vi "Protocol.Command.Main.vi"(8 "Error":errorcluster, 11 "J1939 Main Configuration":T1) -> (0 "error out":errorcluster)   [LabVIEW 2015, in "J1939 Addon Engine.lvlib"]
uses:
  J1939 Addon Engine.lvlib
  Types/Protocol.Configuration.ctl
  <vilib>/NI/NIVS Addon Network Comm/Engine/VeriStand Comm.lvclass
  <vilib>/NI/NIVS Inline Async API/_VS Inline Async API/Process/Process.lvclass
  Types/Protocol.Refs.ctl
  Shared/J1939 Utilities/Types/CAN Outgoing Message Cluster.ctl
  Types/Protocol.RQST Lookup Table Reference.ctl
  Types/Protocol.Address Table Reference.ctl
  Types/Protocol.XNET Settings.ctl
  <vilib>/NI/NIVS Inline Async API/_Data Access Engine/Data Access Engine/Types/Read.DVR.ctl
  <vilib>/NI/NIVS Inline Async API/_Data Access Engine/Access Type Classes/Read/Read.lvclass
  <vilib>/NI/NIVS Inline Async API/_Data Access Engine/Data Access Engine/Types/Write.DVR.ctl
  <vilib>/NI/NIVS Inline Async API/_Data Access Engine/Access Type Classes/Write/Write.lvclass
  Types/Protocol.Command.Commands.ctl
  Types/Protocol.Command.Responses.ctl
  <vilib>/NI/NIVS Inline Async API/_Data Access Engine/Access Type Classes/Read/Read.lvclass/Read.ctl
  <vilib>/NI/NIVS Inline Async API/_Data Access Engine/Access Type Classes/Write/Write.lvclass/Write.ctl
  APIs/Host Automation API/Types/DTC_Action.ctl
  <vilib>/NI/NIVS Inline Async API/_VS Inline Async API/Process/Process.lvclass/Process.ctl
  <vilib>/NI/NIVS Inline Async API/_Data Access Engine/Data Access Engine/Methods/Write.Data.vi
  <vilib>/NI/NIVS Inline Async API/_Data Access Engine/Data Access Engine/Methods/Read.Data.vi
  <vilib>/NI/NIVS Inline Async API/_Data Access Engine/Access Type Classes/Write/Write.ProcessData.vi
  <vilib>/NI/NIVS Inline Async API/_VS Inline Async API/Error Handling Process/SubVIs/Error.ConvertArray.vi
  <vilib>/NI/NIVS Inline Async API/_Data Access Engine/Access Type Classes/Read/Read.ProcessData.vi
  APIs/Host Automation API/J1939 Host Automation API.lvlib
  Shared/J1939 Addon Shared.lvlib
  <vilib>/NI VeriStand/Custom Device Tools/Custom Device Utility Library/Custom Device Utility Library.lvlib
  <vilib>/NI/NIVS Inline Async API/_Data Access Engine/Data Access Engine/Data Access Engine.lvclass
  Shared/J1939 Utilities/J1939 Utilities.lvlib
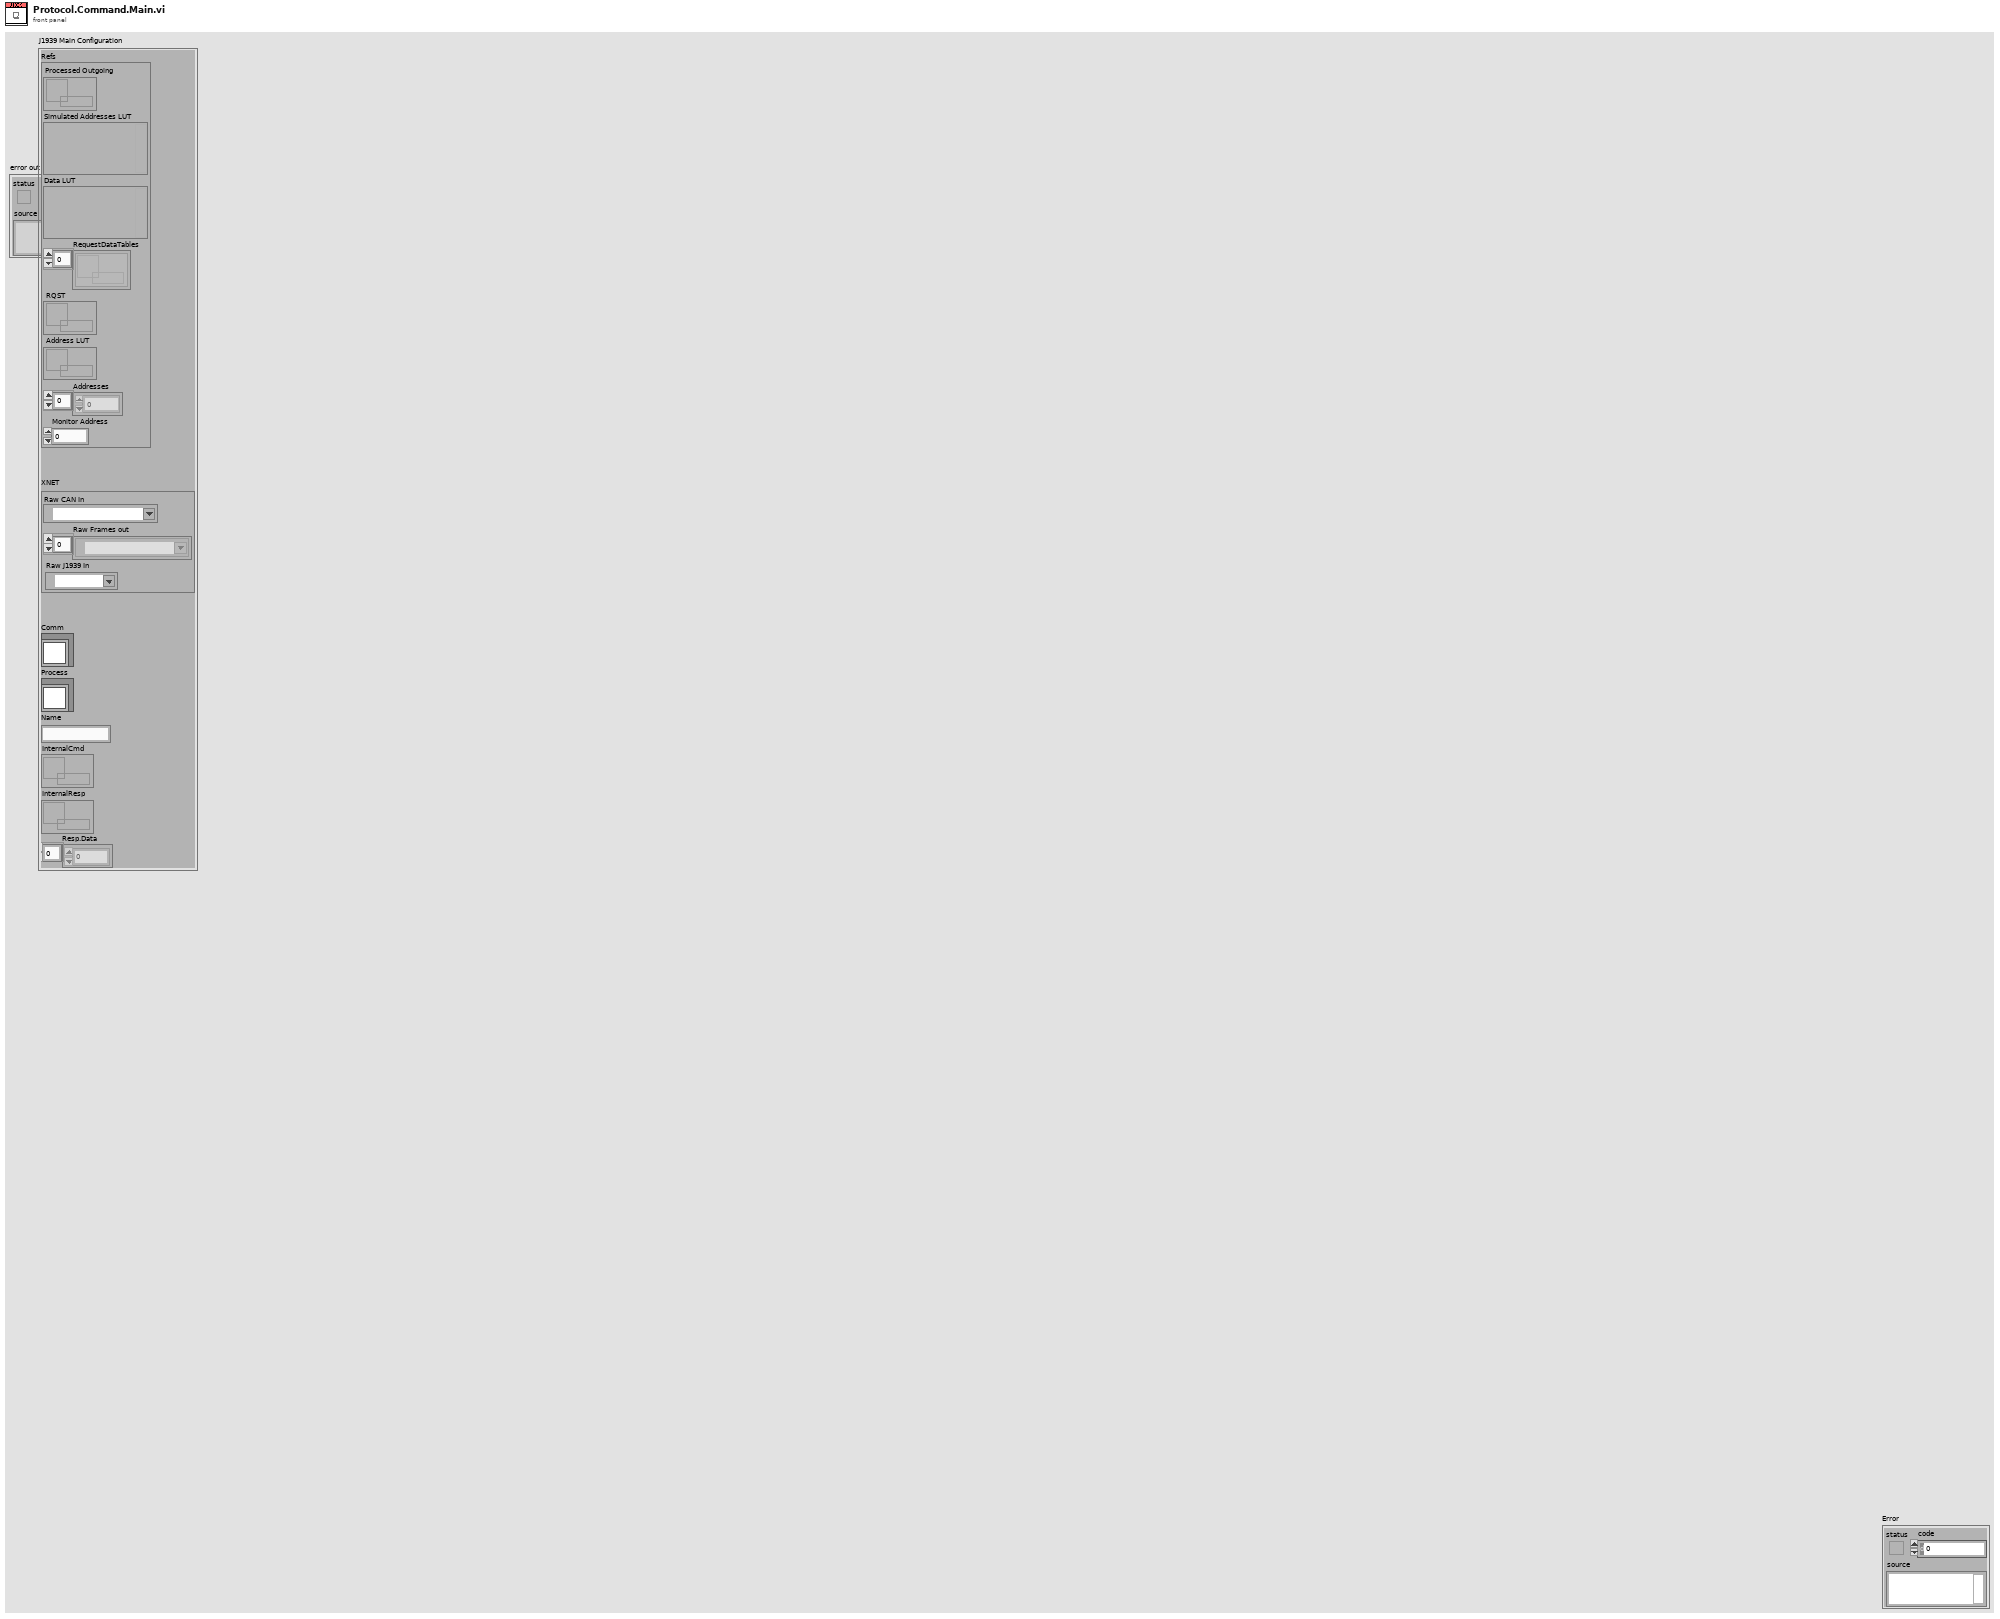
[diagram p1: front panel]
types:
  T1 = typedef "J1939 Addon Engine.lvlib/Protocol.Configuration.ctl" = cluster{"Refs":T2, "XNET":T5, "Comm":refnum<class "VeriStand Comm.lvclass">, "Process":refnum<class "Process.lvclass">, "Name":string, "InternalCmd":T6, "InternalResp":T7, "Resp.Data":dbl[]}
  T2 = typedef "J1939 Addon Engine.lvlib/Protocol.Refs.ctl" = cluster{"Processed Outgoing":refnum<queue>, "Simulated Addresses LUT":variant, "Data LUT":variant, "RequestDataTables":refnum<k33>[], "RQST":T3, "Address LUT":T4, "Addresses":u8[], "Monitor Address":u8}
  T3 = typedef "J1939 Addon Engine.lvlib/Protocol.RQST Lookup Table Reference.ctl" = refnum<data-value>
  T4 = typedef "J1939 Addon Engine.lvlib/Protocol.Address Table Reference.ctl" = refnum<data-value>
  T5 = typedef "J1939 Addon Engine.lvlib/Protocol.XNET Settings.ctl" = cluster{"Raw CAN In":refnum<k21>, "Raw Frames out":refnum<k21>[], "Raw J1939 In":refnum<k21>}
  T6 = typedef "Data Access Engine.lvlib/Data Access Engine.lvclass/Read.DVR.ctl" = refnum<data-value>
  T7 = typedef "Data Access Engine.lvlib/Data Access Engine.lvclass/Write.DVR.ctl" = refnum<data-value>
  T8 = typedef "NI STM.lvlib/TCP Connection Info.ctl" = cluster{"connection ID":refnum<k5>, "meta data":T9[]}
  T9 = typedef "NI STM.lvlib/MetaDataElement.ctl" = string
  T10 = typedef "J1939 Addon Engine.lvlib/Protocol.Command.Responses.ctl" = enum16{"Diagnostic Error Code", "Diagnostic Command Success", "# of DTCs Found", "Request DTC Status"}
  T11 = typedef "J1939 Addon Engine.lvlib/Protocol.Command.Commands.ctl" = enum16{"Diagnostic Command", "Expected DTC", "Address to Query", "DTC Clear Type"}
  T12 = typedef "J1939 Host Automation API.lvlib/DTC_Action.ctl" = enum16{"ALL", "ACTIVE", "INACTIVE"}
  T13 = typedef "J1939 Addon Engine.lvlib/Protocol.Command.States.ctl" = enum8{"Idle", "Refresh Address", "Verify DTCs", "Clear DTCs", "Clear Status Bit", "Clear Error Bit"}
  T14 = typedef "J1939 Host Automation API.lvlib/Verify DTC_Status.ctl" = enum16{"NOT_PRESENT", "ACTIVE", "INACTIVE"}
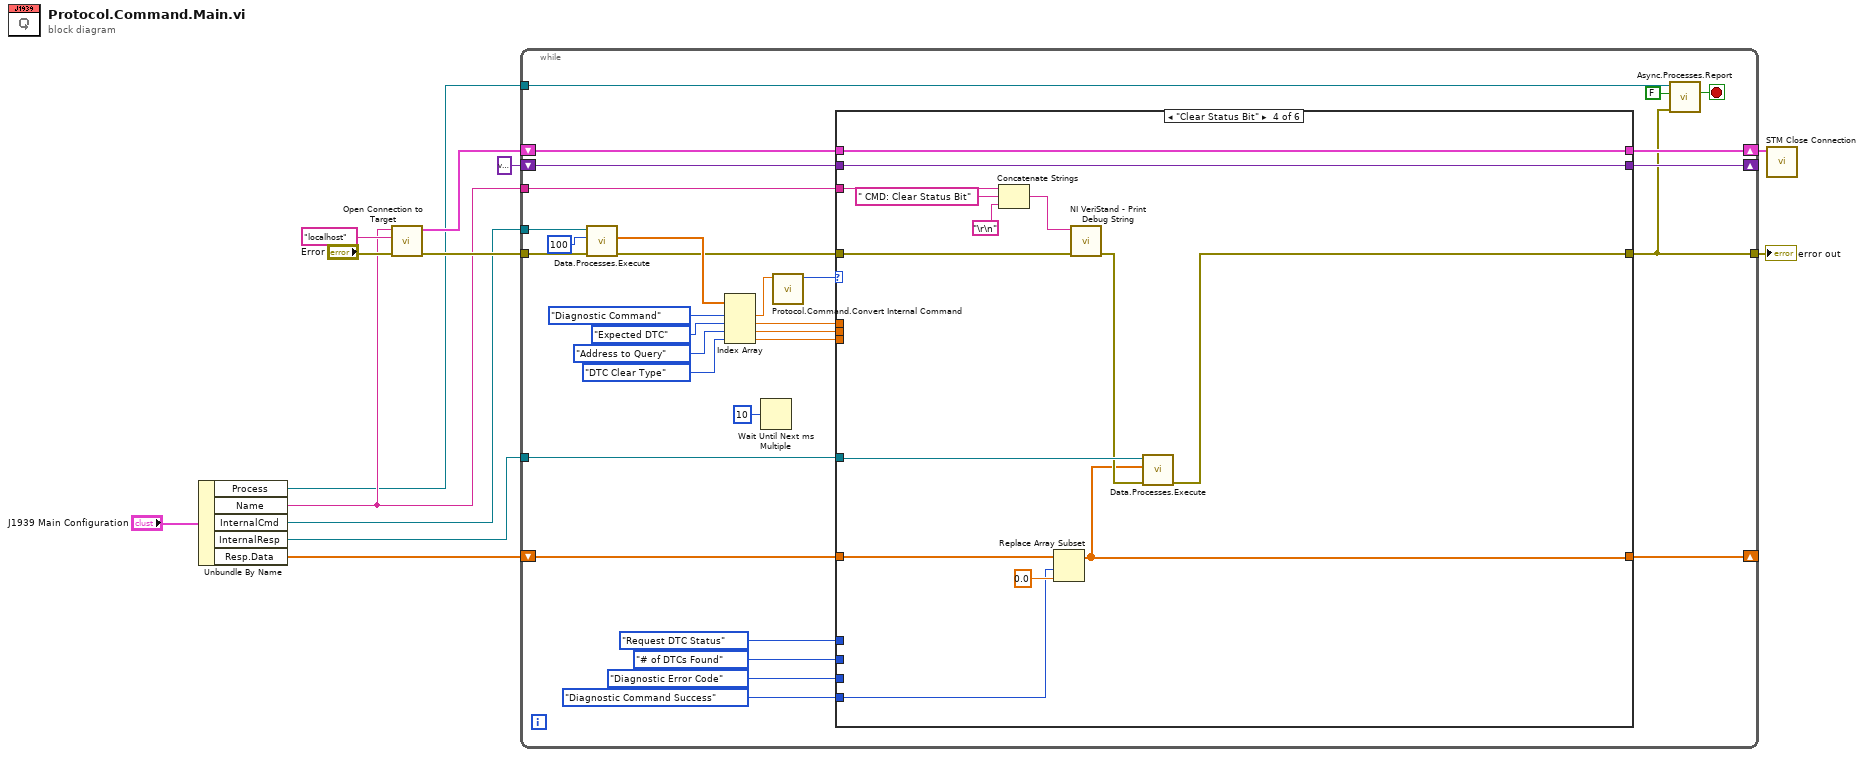
[diagram p0: block diagram]
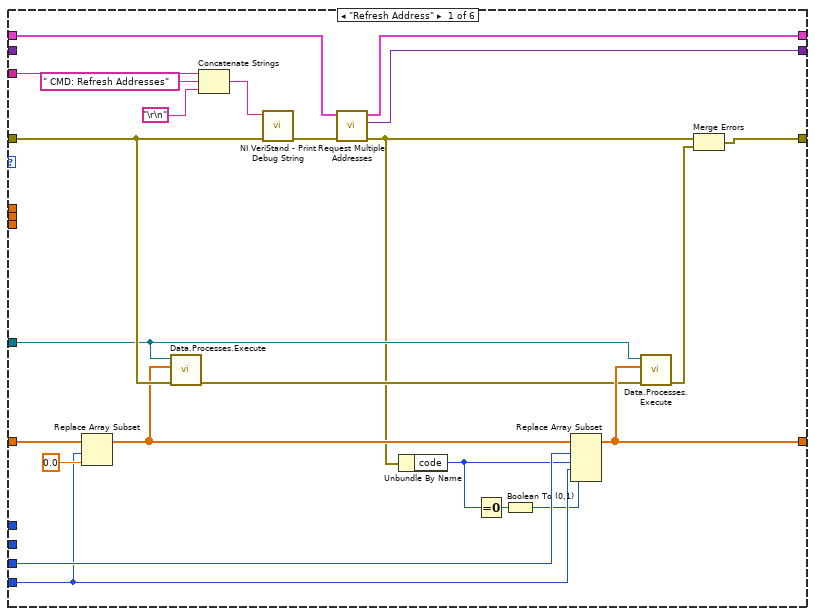
[diagram p2: hidden frame]
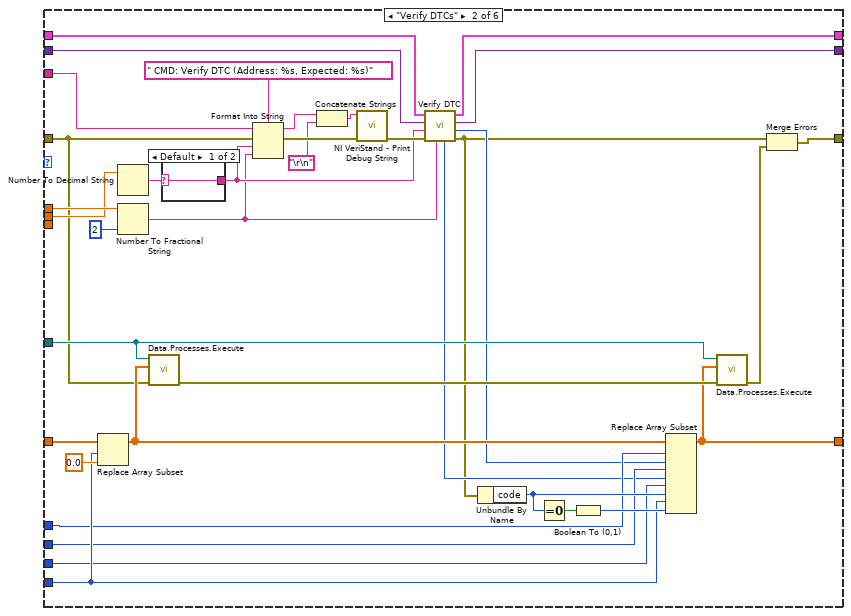
[diagram p3: hidden frame]
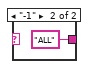
[diagram p4: hidden frame]
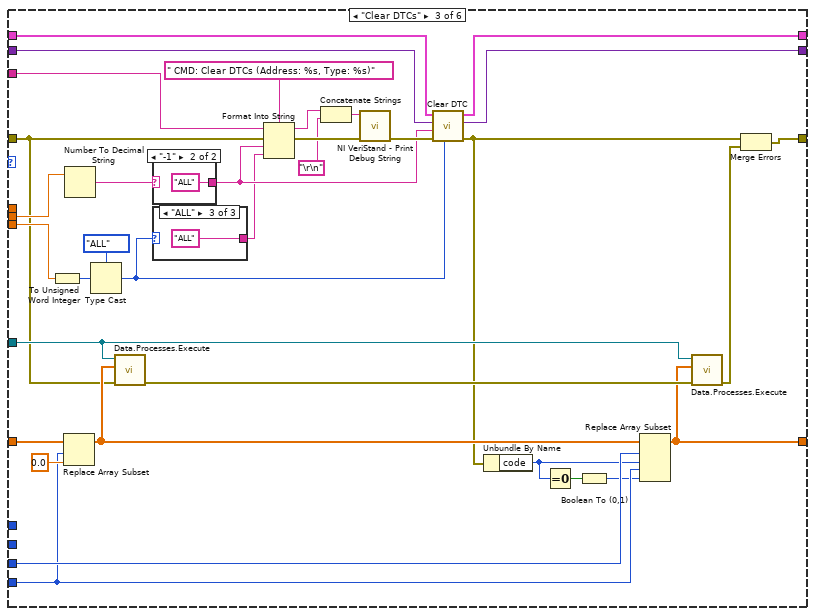
[diagram p5: hidden frame]
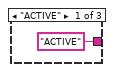
[diagram p6: hidden frame]
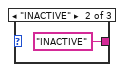
[diagram p7: hidden frame]
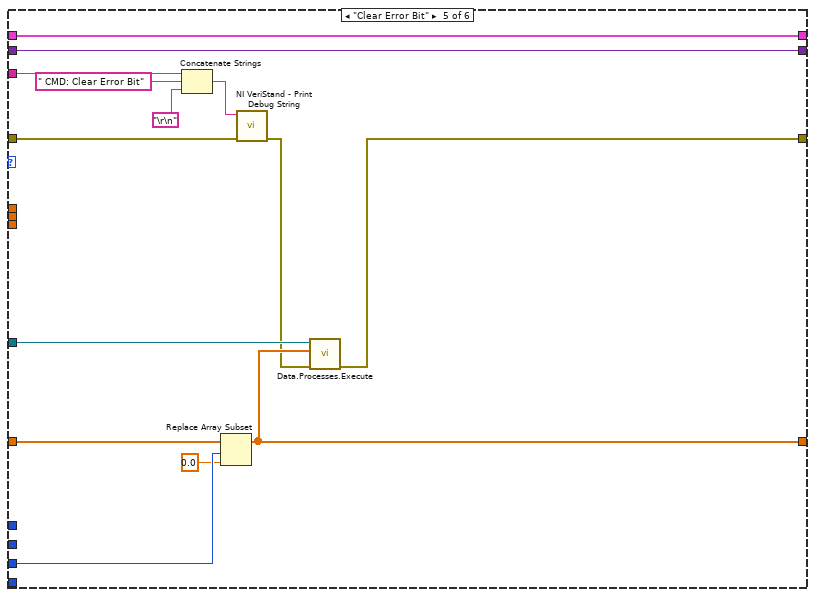
[diagram p9: hidden frame]
diagram:
  n1 = Unbundle By Name("J1939 Main Configuration") -> ("Process"=w3:refnum<class "Process.lvclass">, "Name"=w4:string, "InternalCmd"=w5:T6, "InternalResp"=w6:T7, "Resp.Data"=w1:dbl[])
  n2 = call "Open Connection to Target.vi"("error in (no error)"="Error", "IP Address"="localhost", "TCP Service"=w4) -> ("error out"=w9:errorcluster, "connection info"=w12:T8)  [unwired: 7 in]
  n3 = while {
    shift-right: [w43] -> _
    shift-left: variant ("Address Lookup Table Out") -> [w42]
    shift-right: [w41] -> w10
    shift-left: w12 -> [w44]
    tunnel: [w34] -> w8
    tunnel: w9 -> [w32]
    tunnel: w3 -> [w38]
    tunnel: w4 -> [w37]
    tunnel: w5 -> [w24]
    shift-right: [w17] -> _
    shift-left: w1 -> [w18]
    tunnel: w6 -> [w19]
    stop <- w39 stop-if-true
    n4 = call-poly <vilib>:"Data.Processes.Execute.vi"("error in (no error)"=w32, "timeout ms"=100 ("timeout in ms (0)"), "Ref"=w24) -> ("error out"=w25:errorcluster, "Values"=w31:dbl[])  [unwired: 6 in, 1 out]
    n5 = Index Array(array=w31, index #1=Protocol.Command.Commands."Diagnostic Command" ("Enum"), index #2=Protocol.Command.Commands."Expected DTC" ("Enum"), index #3=Protocol.Command.Commands."Address to Query" ("Enum"), index #4=Protocol.Command.Commands."DTC Clear Type" ("Enum")) -> (element #1=w26:dbl, element #2=w16:dbl, element #3=w15:dbl, element #4=w14:dbl)
    n6 = Wait Until Next ms Multiple(millisecond multiple=u32 10) -> ()  [unwired: 1 out]
    n7 = call "Protocol.Command.Convert Internal Command.vi"("Value"=w26) -> ("Enum"=w35:T13)  [unwired: 9 in, 1 out]
    n8 = case shown="\"Clear Status Bit\"" w35 {
      tunnel: w44 -> [w67 w103 w139 w158 w172 w175]
      tunnel: [w66 w101 w137 w157 w171 w174] -> w43
      tunnel: w42 -> [_ w102 w138 w157 w171 w174]
      tunnel: [w65 w100 w136 w158 w172 w175] -> w41
      tunnel: w25 -> [w59 w80 w106 w156 w170 w176]
      tunnel: [w45 w68 w110 w147 w160 w176] -> w34
      tunnel: w37 -> [w51 w89 w123 w146 w159 _]
      tunnel: Protocol.Command.Responses."Request DTC Status" ("Enum 2") -> [_ w74 _ _ _ _]
      tunnel: Protocol.Command.Responses."# of DTCs Found" ("Enum 2") -> [_ w75 _ _ _ _]
      tunnel: Protocol.Command.Responses."Diagnostic Error Code" ("Enum 2") -> [w56 w76 w116 _ w164 _]
      tunnel: Protocol.Command.Responses."Diagnostic Command Success" ("Enum 2") -> [w55 w77 w115 w149 _ _]
      tunnel: w19 -> [w50 w83 w118 w151 w166 _]
      tunnel: w18 -> [w58 w84 w117 w150 w165 w173]
      tunnel: [w49 w69 w107 w145 w162 w173] -> w17
      tunnel: w16 -> [_ w82 _ _ _ _]
      tunnel: w15 -> [_ w81 w108 _ _ _]
      tunnel: w14 -> [_ _ w109 _ _ _]
      frame "Refresh Address" {
        n9 = Replace Array Subset(array=w58, new element=0.0 ("Value"), index=w55) -> (w57:dbl[])
        n10 = call-poly <vilib>:"Data.Processes.Execute.vi"("error in (no error)"=w59, "Values"=w57, "Ref"=w50) -> ("error out"=w48:errorcluster)  [unwired: 8 in]
        n11 = Concatenate Strings(w51, " CMD: Refresh Addresses" ("string"), "\r\n") -> (w62:string)
        n12 = call <vilib>:"NI VeriStand - Print Debug String.vi"("error in (no error)"=w59, "Message"=w62) -> ("error out"=w52:errorcluster)  [unwired: 9 in]
        n13 = call "Request Multiple Addresses.vi"("error in (no error)"=w52, "connection info"=w67) -> ("error out"=w47:errorcluster, "variant"=w66:variant, "connection info"=w65:T8)  [unwired: 6 in, 1 out]
        n14 = Unbundle By Name(w47) -> ("code"=w53:i32)
        n15 = Equal To 0?(x=w53) -> (x = 0?=w64:bool)
        n16 = Boolean To (0,1)(Boolean=w64) -> (0, 1=w54:i16)
        n17 = Replace Array Subset(array=w57, new element #1=w53, index #1=w56, new element #2=w54, index #2=w55) -> (w49:dbl[])
        n18 = call-poly <vilib>:"Data.Processes.Execute.vi"("error in (no error)"=w48, "Values"=w49, "Ref"=w50) -> ("error out"=w46:errorcluster)  [unwired: 8 in]
        n19 = Merge Errors(w47, w46) -> (w45:errorcluster)
      }
      frame "Verify DTCs" {
        n20 = Replace Array Subset(array=w84, new element=0.0 ("Value"), index=w77) -> (w86:dbl[])
        n21 = Number To Decimal String(number=w81) -> (decimal integer string=w99:string)  [unwired: 1 in]
        n22 = Number To Fractional String(number=w82, precision (6)=i16 2) -> (F-format string=w92:string)  [unwired: 2 in]
        n23 = call-poly <vilib>:"Data.Processes.Execute.vi"("error in (no error)"=w80, "Values"=w86, "Ref"=w83) -> ("error out"=w85:errorcluster)  [unwired: 8 in]
        n24 = case shown="Default" w99 {
          selector: w99 -> [w104 _]
          tunnel: [w104 "ALL"] -> w93
          frame Default {
          }
          frame "-1" {
          }
        }
        n25 = Format Into String(format string=" CMD: Verify DTC (Address: %s, Expected: %s)" ("string"), initial string=w89, error in=w80, w93, w92) -> (resulting string=w96:string, error out=w95:errorcluster)
        n26 = Concatenate Strings(w96, "\r\n") -> (w91:string)
        n27 = call <vilib>:"NI VeriStand - Print Debug String.vi"("error in (no error)"=w95, "Message"=w91) -> ("error out"=w94:errorcluster)  [unwired: 9 in]
        n28 = call "Verify DTC.vi"("Expected DTC"=w92, "error in"=w94, "Address"=w93, "Address Lookup Table"=w102, "connection info"=w103) -> ("error out"=w71:errorcluster, "Status"=w73:T14, "Address Lookup Table Out"=w101:variant, "connection info"=w100:T8, "Found DTCs"=w72:i32)  [unwired: 2 in]
        n29 = Unbundle By Name(w71) -> ("code"=w78:i32)
        n30 = Equal To 0?(x=w78) -> (x = 0?=w88:bool)
        n31 = Boolean To (0,1)(Boolean=w88) -> (0, 1=w79:i16)
        n32 = Replace Array Subset(array=w86, new element #1=w73, index #1=w74, new element #2=w72, index #2=w75, new element #3=w78, index #3=w76, new element #4=w79, index #4=w77) -> (w69:dbl[])
        n33 = call-poly <vilib>:"Data.Processes.Execute.vi"("error in (no error)"=w85, "Values"=w69, "Ref"=w83) -> ("error out"=w70:errorcluster)  [unwired: 8 in]
        n34 = Merge Errors(w71, w70) -> (w68:errorcluster)
      }
      frame "Clear DTCs" {
        n35 = To Unsigned Word Integer(number=w109) -> (unsigned 16bit integer=w134:u16)
        n36 = Replace Array Subset(array=w117, new element=0.0 ("Value"), index=w115) -> (w120:dbl[])
        n37 = Number To Decimal String(number=w108) -> (decimal integer string=w135:string)  [unwired: 1 in]
        n38 = Type Cast(type=DTC_Action."ALL" ("Action"), x=w134) -> (*(type *) &x=w131:T12)
        n39 = call-poly <vilib>:"Data.Processes.Execute.vi"("error in (no error)"=w106, "Values"=w120, "Ref"=w118) -> ("error out"=w119:errorcluster)  [unwired: 8 in]
        n40 = case shown="\"-1\"" w135 {
          selector: w135 -> [w143 _]
          tunnel: [w143 "ALL"] -> w128
          frame Default {
          }
          frame "-1" {
          }
        }
        n41 = case shown="\"ALL\"" w131 {
          tunnel: ["ACTIVE" "INACTIVE" "ALL"] -> w127
          frame "ACTIVE" {
          }
          frame "INACTIVE" {
          }
          frame "ALL" {
          }
        }
        n42 = Format Into String(format string=" CMD: Clear DTCs (Address: %s, Type: %s)" ("string"), initial string=w123, error in=w106, w128, w127) -> (resulting string=w125:string, error out=w130:errorcluster)
        n43 = Concatenate Strings(w125, "\r\n") -> (w124:string)
        n44 = call <vilib>:"NI VeriStand - Print Debug String.vi"("error in (no error)"=w130, "Message"=w124) -> ("error out"=w129:errorcluster)  [unwired: 9 in]
        n45 = call "Clear DTC.vi"("Action"=w131, "error in"=w129, "Address (ALL)"=w128, "Address Lookup Table"=w138, "connection info"=w139) -> ("error out"=w111:errorcluster, "Address Lookup Table Out"=w137:variant, "connection info"=w136:T8)  [unwired: 4 in]
        n46 = Unbundle By Name(w111) -> ("code"=w113:i32)
        n47 = Equal To 0?(x=w113) -> (x = 0?=w122:bool)
        n48 = Boolean To (0,1)(Boolean=w122) -> (0, 1=w114:i16)
        n49 = Replace Array Subset(array=w120, new element #1=w113, index #1=w116, new element #2=w114, index #2=w115) -> (w107:dbl[])
        n50 = call-poly <vilib>:"Data.Processes.Execute.vi"("error in (no error)"=w119, "Values"=w107, "Ref"=w118) -> ("error out"=w112:errorcluster)  [unwired: 8 in]
        n51 = Merge Errors(w111, w112) -> (w110:errorcluster)
      }
      frame "Clear Status Bit" {
        n52 = Concatenate Strings(w146, " CMD: Clear Status Bit" ("string"), "\r\n") -> (w154:string)
        n53 = Replace Array Subset(array=w150, new element=0.0 ("Value"), index=w149) -> (w145:dbl[])
        n54 = call <vilib>:"NI VeriStand - Print Debug String.vi"("error in (no error)"=w156, "Message"=w154) -> ("error out"=w148:errorcluster)  [unwired: 9 in]
        n55 = call-poly <vilib>:"Data.Processes.Execute.vi"("error in (no error)"=w148, "Values"=w145, "Ref"=w151) -> ("error out"=w147:errorcluster)  [unwired: 8 in]
      }
      frame "Clear Error Bit" {
        n56 = Concatenate Strings(w159, " CMD: Clear Error Bit" ("string"), "\r\n") -> (w168:string)
        n57 = Replace Array Subset(array=w165, new element=0.0 ("Value"), index=w164) -> (w162:dbl[])
        n58 = call <vilib>:"NI VeriStand - Print Debug String.vi"("error in (no error)"=w170, "Message"=w168) -> ("error out"=w161:errorcluster)  [unwired: 9 in]
        n59 = call-poly <vilib>:"Data.Processes.Execute.vi"("error in (no error)"=w161, "Values"=w162, "Ref"=w166) -> ("error out"=w160:errorcluster)  [unwired: 8 in]
      }
      frame "Idle" {
      }
    }
    n60 = call <vilib>:"Async.Processes.Report.vi"("Error"=w34, "Stop Async on Error?"=FALSE ("Stop on Error?"), "Process in"=w38) -> ("Stop"=w39:bool)  [unwired: 7 in, 1 out]
  }
  "error out" <- w8
  n61 = call "STM Close Connection.vi"("connection info"=w10) -> ()  [unwired: 10 in, 1 out]
